vi "Write combo box ctrl values to initial values section.vi"(6 "Index of property keys":i32[](array[numeric]), 9 "Cancelled":bool, 11 "Combo box ref":refnum<vi>) -> (0 "error out":errorcluster)   [LabVIEW 2020]
uses:
  Typedefs/Which path.ctl
  <vilib>/Utility/config.llb/NI_LVConfig.lvlib
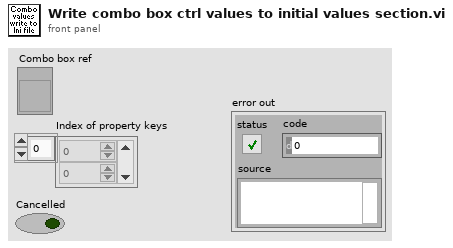
[diagram p1: front panel]
types:
  T1 = typedef "Which path.ctl" = enum16{"Configuration Files", "Calibration Files", "Images", "Setup.ini", "Loaded User profile.ini", "User's-Previous session.ini", "New user profile.ini", "Selected User profile.ini", "User profiles folder", "Power meter scaling.txt", "FOV Cal.ini", "Calibration.ini"}
  T2 = typedef "NI_LVConfig.lvlib/Config Data RefNum.ctl" = refnum<k1>
  T3 = typedef "Ini file interface (String).ctl" = cluster{"key":string, "Save?":bool, "Default":string}[]
  T4 = cluster{"key":string, "Save?":bool, "Default":string}
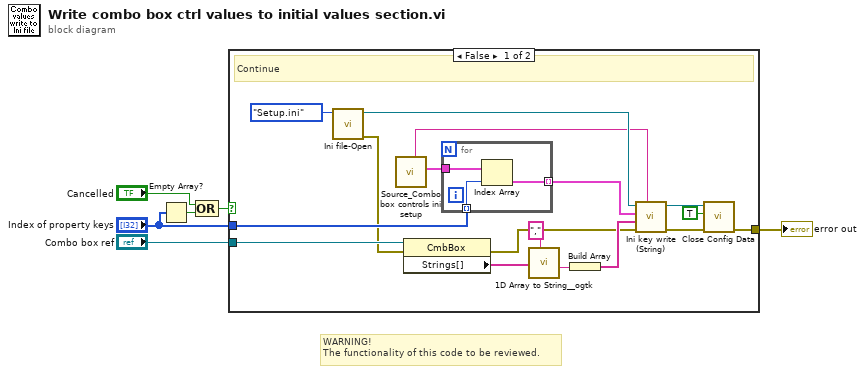
[diagram p0: block diagram]
diagram:
  # "WARNING!\nThe functionality of this code to be reviewed."
  n1 = Empty Array?(array="Index of property keys") -> (empty?=w3:bool)
  n2 = Compound Arithmetic op=OR("Cancelled", w3) -> (w1:bool)
  n3 = case shown="False" w1 {
    tunnel: "Combo box ref" -> [w22 _]
    tunnel: "Index of property keys" -> [w21 _]
    tunnel: [w16 _] -> w6
    frame False {
      # "Continue"
      n4 = call "Ini file-Open.vi"("Which file?"=Which_path."Setup.ini") -> ("error out"=w14:errorcluster, "User profile ini file ref"=w10:T2)  [unwired: 7 in, 2 out]
      n5 = call "Source_Combo box controls ini setup.vi"() -> ("Keys setup"=w23:T3, "Section name"=w8:string)  [unwired: 9 in, 1 out]
      n6 = property class="CmbBox"(reference=w22, error in=w14) -> (error out=w12:errorcluster, "Strings[]"=w20:string[])  [unwired: 1 out]
      n7 = for {
        tunnel: w23 -> [w26]
        tunnel: [w25] -> w7 mode=indexing
        tunnel: w21 -> [w24] mode=indexing
        n8 = Index Array(array=w26, index=w24) -> (element=w25:T4)
      }
      n9 = call <userlib>:"1D Array to String__ogtk.vi"("delimiter (Tab)"=",", "Array of Strings"=w20) -> ("delimited string"=w18:string)  [unwired: 9 in]
      n10 = Build Array(w18) -> (w13:string[])
      n11 = call "Ini key write (String).vi"("Section"=w8, "error in (no error)"=w12, "Values (String)"=w13, "Ini file interface"=w7, "Ini file refnum in"=w10) -> ("error out"=w11:errorcluster, "Ini file refnum out"=w9:T2)  [unwired: 5 in]
      n12 = call <vilib>:"Close Config Data.vi"("error in (no error)"=w11, "write file if changed (T)"=TRUE, "refnum"=w9) -> ("error out"=w16:errorcluster)  [unwired: 7 in, 1 out]
    }
    frame True {
      # "Cancelled or Empty keys array"
    }
  }
  "error out" <- w6
